vi "Shutdown State Machine Loop.vi"() -> ()   [LabVIEW 2015]
uses:
  Shutdown State Machine.lvsc/State.ctl
  Shutdown State Machine.lvsc/Inputs.ctl
  Shutdown State Machine.lvsc/StatechartState.ctl
  Shutdown State Machine.lvsc/CompanionDiagram.vi/7/SC Main.vi
  Shutdown State Machine.lvsc/CompanionDiagram.vi/7/Upd State.vi
  Shutdown State Machine.lvsc/CompanionDiagram.vi/7/Trans Graph0.vi
  Shutdown State Machine.lvsc/CompanionDiagram.vi/7/EnterGraphCore.vi
  <vilib>/FPGAPlugInAG/sbRIO-9627/niLvFpga_Open_sbRIO-9627.vi
  Global Data.vi
  <vilib>/Utility/error.llb/Error Cluster From Error Code.vi
  <vilib>/rvi/errors/niLvFpgaAdjustHostInterfaceError.vi
  Shutdown State Machine.lvsc/CompanionDiagram.vi
  <vilib>/FPGAPlugInAG/sbRIO-9627/niLvFpga_Close_sbRIO-9627.vi
  <vilib>/rvi/interface/nirviOpenFPGA/nirviOpenFPGA.xnode
  FPGA Bitfiles/Latest.lvbitx
  Shutdown State Machine.lvsc/Trigger.ctl
  <vilib>/rvi/interface/nirviReadWriteControl/nirviReadWriteControl.xnode
  <vilib>/Statechart/Infrastructure/RTStatechart/RunTime SCN.xnode
  Shutdown State Machine.lvsc/Outputs.ctl
  AIR Status.ctl
  Shutdown State Machine.lvsc
  <vilib>/rvi/interface/nirviCloseFPGA/nirviCloseFPGA.xnode
  NiFpgaLv.dll
panel:
  out "Shutdown State":T1=enum."TSMS Off"
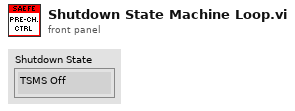
[diagram p1: front panel]
types:
  T1 = typedef "Shutdown State Machine.lvsc/State.ctl" = enum16{"NI.SC.Initial", "NI.SC.History", "NI.SC.ShallowHistory", "NI.SC.Terminal", "Coolant Pump Started/AIR's On", "AIRs On", "Precharge", "TSMS Off"}
  T2 = typedef "Shutdown State Machine.lvsc/Inputs.ctl" = cluster{"TSMS Status In":bool, "Precharge Time":u32}
  T3 = typedef "Shutdown State Machine.lvsc/Outputs.ctl" = cluster{"Positive AIR Enable":bool, "AIR Status":T4, "Coolant Pump":bool, "Precharge Failed":bool, "bDCDCDisable":bool}
  T4 = typedef "AIR Status.ctl" = enum16{"Off", "Precharge", "On"}
  T5 = typedef "Shutdown State Machine.lvsc/StatechartState.ctl" = T1[]
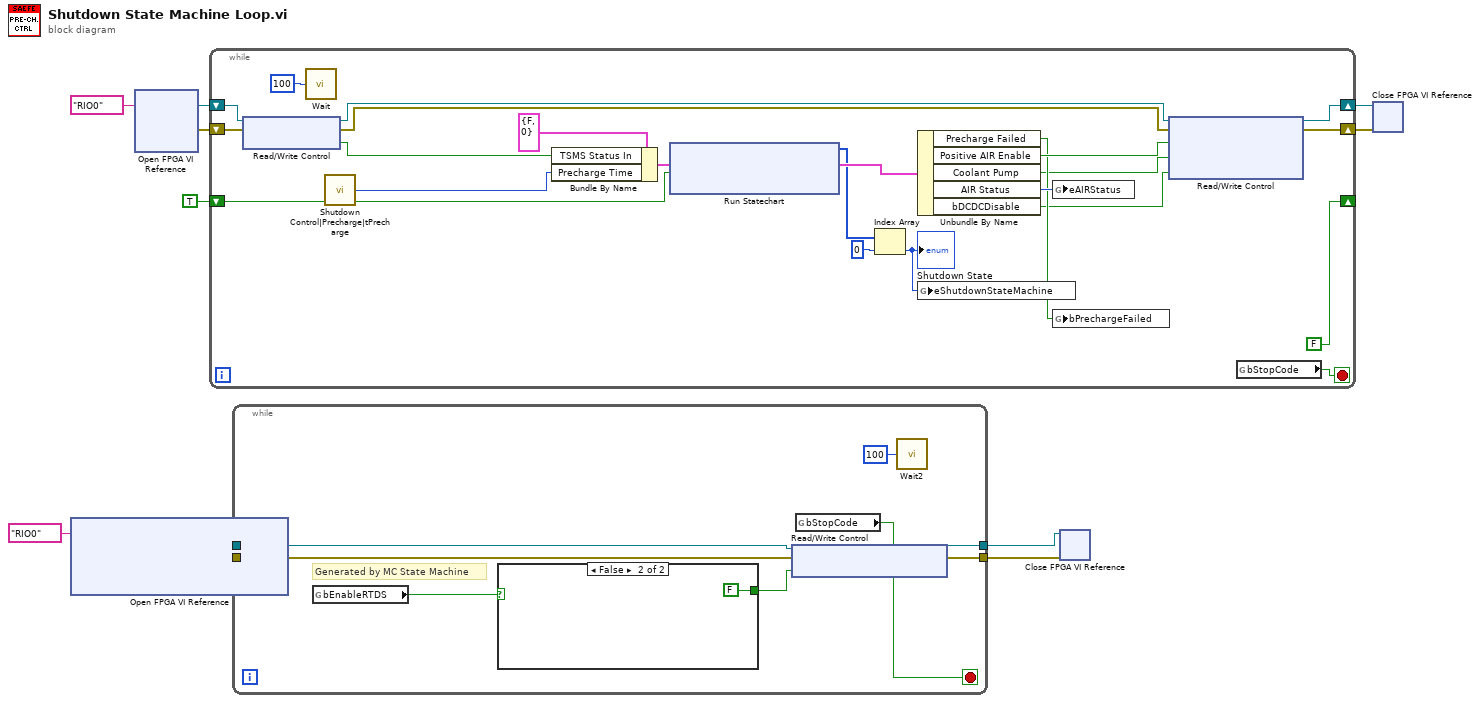
[diagram p0: block diagram]
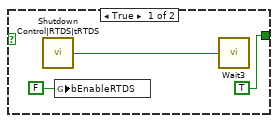
[diagram p2: hidden frame]
diagram:
  n1 = xnode "Open FPGA VI Reference"("resource name"=tag "RIO0") -> ("FPGA VI Reference Out"=w7:refnum<k20>, "error out"=w6:errorcluster)  [unwired: 1 in]
  n2 = xnode "Open FPGA VI Reference"("resource name"=tag "RIO0") -> ("FPGA VI Reference Out"=w11:refnum<k20>, "error out"=w10:errorcluster)  [unwired: 1 in]
  n3 = while {
    shift-right: [FALSE] -> _
    shift-left: TRUE -> [w29]
    shift-right: [w17] -> w4
    shift-left: w11 -> [w34]
    shift-right: [w16] -> w3
    shift-left: w10 -> [w33]
    stop <- w19 stop-if-true
    n4 = xnode "Read/Write Control"("FPGA VI Reference In"=w34, "error in"=w33) -> ("FPGA VI Reference Out"=w31:refnum<k20>, "error out"=w30:errorcluster, "bTSMSInStatus"=w25:bool)
    n5 = call "Wait"("Count(mSec)"=u32 100) -> ()  [unwired: 1 out]
    n6 = call "Shutdown Control|Precharge|tPrecharge"() -> ("Value"=w14:u32)
    n7 = Bundle By Name(cluster=T2 {"TSMS Status In"=FALSE, "Precharge Time"=0} ("Inputs"), "TSMS Status In"=w25, "Precharge Time"=w14) -> (w26:T2)
    n8 = xnode "Run Statechart"("Init?"=w29, "Inputs"=w26) -> ("Outputs"=w24:T3, "Active States"=w23:T5)  [unwired: 1 in, 1 out]
    n9 = Index Array(array=w23, index=0) -> (element=w21:T1)
    "Shutdown State" <- w21
    n10 = Unbundle By Name(w24) -> ("Precharge Failed"=w15:bool, "Positive AIR Enable"=w18:bool, "Coolant Pump"=w13:bool, "AIR Status"=w20:T4, "bDCDCDisable"=w12:bool)
    n11 = global write "Global Data.vi" "eShutdownStateMachine"(w21) -> ()
    n12 = global write "Global Data.vi" "eAIRStatus"(w20) -> ()
    n13 = global write "Global Data.vi" "bPrechargeFailed"(w15) -> ()
    n14 = xnode "Read/Write Control"("FPGA VI Reference In"=w31, "error in"=w30, "bPosAIREnable"=w18, "bCoolantPumpEnable"=w13, "bDCDCDisable"=w12) -> ("FPGA VI Reference Out"=w17:refnum<k20>, "error out"=w16:errorcluster)
    n15 = global read "Global Data.vi" "bStopCode"() -> (w19:bool)
  }
  n16 = while {
    tunnel: [w77] -> w9
    tunnel: [w76] -> w8
    tunnel: w7 -> [w75]
    tunnel: w6 -> [w74]
    stop <- w73 stop-if-true
    # "Generated by MC State Machine"
    n17 = global read "Global Data.vi" "bEnableRTDS"() -> (w78:bool)
    n18 = case shown="False" w78 {
      tunnel: [TRUE FALSE] -> w72
      frame True {
        n19 = call "Shutdown Control|RTDS|tRTDS"() -> ("Value"=w80:u32)
        n20 = global write "Global Data.vi" "bEnableRTDS"(FALSE ("Make Sound?")) -> ()
        n21 = call "Wait3"("Count(mSec)"=w80) -> ()  [unwired: 1 out]
      }
      frame False {
      }
    }
    n22 = xnode "Read/Write Control"("FPGA VI Reference In"=w75, "error in"=w74, "bRTDSEnable"=w72) -> ("FPGA VI Reference Out"=w77:refnum<k20>, "error out"=w76:errorcluster)
    n23 = global read "Global Data.vi" "bStopCode"() -> (w73:bool)
    n24 = call "Wait2"("Count(mSec)"=u32 100) -> ()  [unwired: 1 out]
  }
  n25 = xnode "Close FPGA VI Reference"("FPGA VI Reference In"=w9, "error in"=w8) -> ()  [unwired: 1 out]
  n26 = xnode "Close FPGA VI Reference"("FPGA VI Reference In"=w4, "error in"=w3) -> ()  [unwired: 1 out]
